vi "Factory.vi"(0 "TTLControlledDevice in":refnum<class "TTLControlledDevice.lvclass">, 7 "Variant":variant, 9 "Prefix":string, 11 "error in (no error)":errorcluster) -> (4 "TTLControlledDevice out":refnum<class "TTLControlledDevice.lvclass">, 8 "Type":string, 15 "error out":errorcluster)   [LabVIEW 2020, in "TTLControlledDevice.lvclass"]
uses:
  TTLControlledDevice.lvclass
  epl-vi-lib/Koop/KObject Class/KObject.lvclass
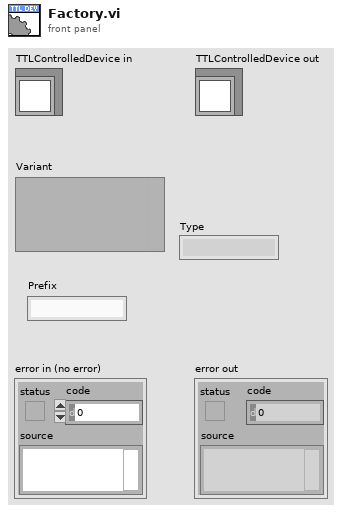
[diagram p1: front panel]
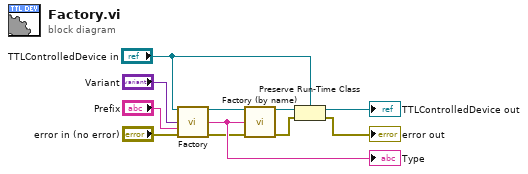
[diagram p0: block diagram]
diagram:
  n1 = call-parent "Factory.vi"("KObject in"="TTLControlledDevice in", "Variant"="Variant", "Prefix"="Prefix", "error in (no error)"="error in (no error)") -> ("KObject out"=w8:refnum<class "TTLControlledDevice.lvclass">, "Type"=w7:string, "error out"=w6:errorcluster)  [unwired: 9 in]
  "Type" <- w7
  n2 = call "Factory (by name).vi"("TTLDevice in"=w8, "Class Name"=w7, "error in (no error)"=w6) -> ("TTLDevice out"=w4:refnum<class "TTLControlledDevice.lvclass">, "error out"=w5:errorcluster)  [unwired: 11 in]
  n3 = Preserve Run-Time Class(object in=w4, error in=w5, 2:"TTLControlledDevice in") -> (object out=→"TTLControlledDevice out":refnum<class "TTLControlledDevice.lvclass">, error out=→"error out":errorcluster)
